vi "Parse CSV From cRIO (Mark Siekmeier's conflicted copy 2013-04-30).vi"(0 "/path/":string="/auton/", 1 "File Name":string, 4 "Header Row?":bool=TRUE) -> (5 "Output Array":dbl[][](array[numeric]))   [LabVIEW 2012]
uses:
  <vilib>/Utility/file.llb/Read From Spreadsheet File (string).vi
panel:
  out "Path and file":string
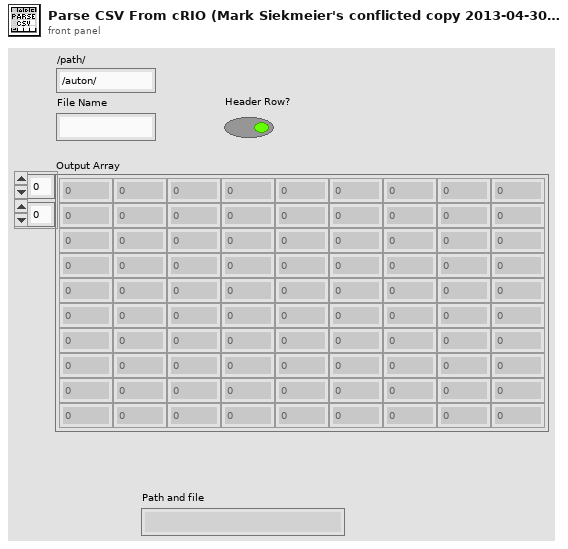
[diagram p1: front panel]
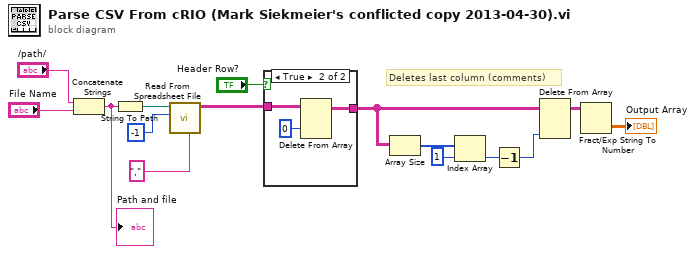
[diagram p0: block diagram]
diagram:
  # "Deletes last column (comments)"
  n1 = Concatenate Strings("/path/", "File Name") -> (w11:string)
  "Path and file" <- w11
  n2 = String To Path(string=w11) -> (path=w10:path)
  n3 = call-poly <vilib>:"Read From Spreadsheet File.vi"("delimiter (\\t)"="," ("delimiter (\\t)"), "number of rows (all:-1)"=-1, "file path (dialog if empty)"=w10) -> ("all rows"=w9:string[][])  [unwired: 2 in, 6 out]
  n4 = case shown="True" "Header Row?" {
    tunnel: w9 -> [w16 w19]
    tunnel: [w16 w17] -> w3
    frame False {
    }
    frame True {
      n5 = Delete From Array(array=w19, index (row)=0) -> (array with subset deleted=w17:string[][])  [unwired: 2 in, 1 out]
    }
  }
  n6 = Array Size(array=w3) -> (size(s)=w7:i32[])
  n7 = Index Array "Index Array"(array=w7, index=1) -> (element=w5:i32)
  n8 = Decrement(x=w5) -> (x-1=w4:i32)
  n9 = Delete From Array(array=w3, index (col)=w4) -> (array with subset deleted=w2:string[][])  [unwired: 2 in, 1 out]
  n10 = Fract/Exp String To Number(string=w2) -> (number=→"Output Array":dbl[][])  [unwired: 3 in, 1 out]
